vi "counter-state-machine.vi"() -> ()   [LabVIEW 2025]
panel:
  out "Count":string
  in  "Decrease":bool
  in  "Increase":bool
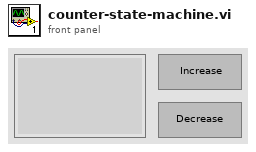
[diagram p1: front panel]
types:
  T1 = enum16{"Waiting For Event", "Increase", "Decrease"}
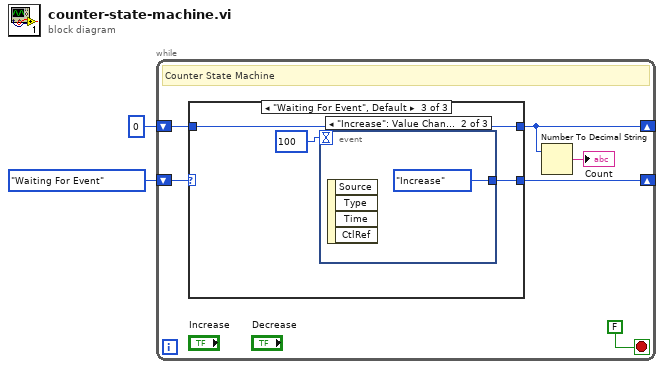
[diagram p0: block diagram]
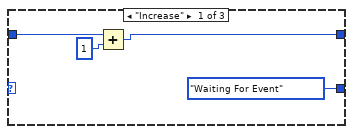
[diagram p2: hidden frame]
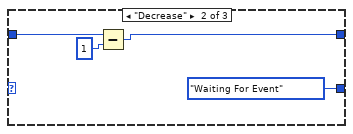
[diagram p3: hidden frame]
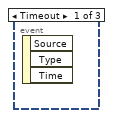
[diagram p4: hidden frame]
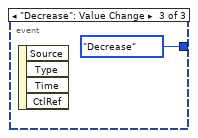
[diagram p5: hidden frame]
diagram:
  n1 = while {
    shift-right: [w6] -> _
    shift-left: T1."Waiting For Event" -> [w8]
    shift-right: [w5] -> _
    shift-left: 0 -> [w7]
    stop <- FALSE stop-if-true
    # "Counter State Machine"
    n2 = case shown="\"Waiting For Event\", Default" w8 {
      tunnel: [w10 w14 w17] -> w5
      tunnel: w7 -> [w12 w16 w17]
      tunnel: [T1."Waiting For Event" T1."Waiting For Event" w18] -> w6
      frame "Increase" {
        n3 = Add(x=w12, y=1) -> (x+y=w10:i32)
      }
      frame "Decrease" {
        n4 = Subtract(x=w16, y=1) -> (x-y=w14:i32)
      }
      frame "Waiting For Event", Default {
        n5 = event shown="[1] \"Increase\": Value Change" {
          selector: _ -> [_ _ _]
          dyn-events: _ -> [_ _ _]
          timeout: 100 -> [_ _ _]
          tunnel: [_ T1."Increase" T1."Decrease"] -> w18
          event Timeout {
            n6 = event-data() -> ()  [unwired: 1 in, 3 out]
          }
          event "Increase": Value Change {
            n7 = event-data() -> ()  [unwired: 1 in, 4 out]
          }
          event "Decrease": Value Change {
            n8 = event-data() -> ()  [unwired: 1 in, 4 out]
          }
        }
      }
    }
    n9 = Number To Decimal String(number=w5) -> (decimal integer string=→"Count":string)  [unwired: 1 in]
  }
